vi "Pockels Cal-Write meas AI to sys config.vi"(8 "error in (no error)":errorcluster) -> (0 "error out":errorcluster)   [LabVIEW 2013]
uses:
  Typedefs/HW config states enum.ctl
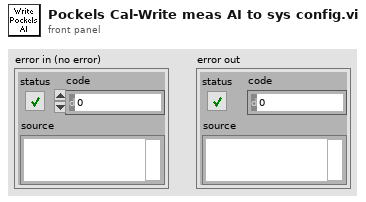
[diagram p1: front panel]
types:
  T1 = typedef "HW config states enum.ctl" = enum16{"Load from file", "Save to file", "Write all", "Read all", "Write XY stage settings", "Write DAQ FPGA settings", "Write Control FPGA settings", "Write Phys Channels", "Clear", "Compare from file"}
  T2 = typedef "Sys Configuration.ctl" = cluster{"XY Stage":T3, "DAQ FPGA":T4, "Control system":T8, "Encoder":T9, "DAQmx Chan":T10, "Computer MAC address":string, "Cam VidRec":T11, "Externalise Triggers":bool, "Laser wavelength (nm)":dbl}
  T3 = typedef "XY Stage config cluster.ctl" = cluster{"COM port":refnum<visa-resource-name>, "XY stage available":bool}
  T4 = typedef "DAQ FPGA config cluster.ctl" = cluster{"Ref":T5, "Target":T6, "Clock Freq (MHz) ":dbl, "input card type":T7, "Samples Wait after Trigger":u16, "AOD fill":u16, "StartupDelay":i32, "Slip Cycle (clock cycles)":u32, "Add Cycle":bool}
  T5 = typedef "FPGA Ref.ctl" = refnum<k20>
  T6 = typedef "nirio_resource_hc.ctl" = tag
  T7 = typedef "FPGA input type AC-DC.ctl" = enum16{"AC Card", "DC Card"}
  T8 = typedef "CTRL system config cluster.ctl" = cluster{"Ethernet opened":bool, "Ethernet Port":u32, "Ctrl FPGA available":bool, "Ctrl FPGA Clock (MHz)":dbl, "Ctrl system MAC address":string, "Control system.Network adapter name":string, "AOD 1 Amplitude":i16, "AOD 2 Amplitude":i16, "AOD 3 Amplitude":i16, "AOD 4 Amplitude":i16, "Data Time Interval (ns)":dbl, "T0 (ns)":dbl, "Ta (ns)":dbl}
  T9 = typedef "Encoder config cluster.ctl" = cluster{"IP address":string, "Port":u16, "Encoder available":bool, "Wheel radius (cm)":dbl}
  T10 = typedef "DAQmx physical channels cluster.ctl" = cluster{"Pockels AO":tag, "Hard shutter AO":tag, "PMT AOs":tag, "Power meter AI":tag}
  T11 = typedef "Cam VidRec HW config setup cluster.ctl" = cluster{"DO flag-Video record":tag, "DO flag-Trial start":tag, "VidRec available":bool}
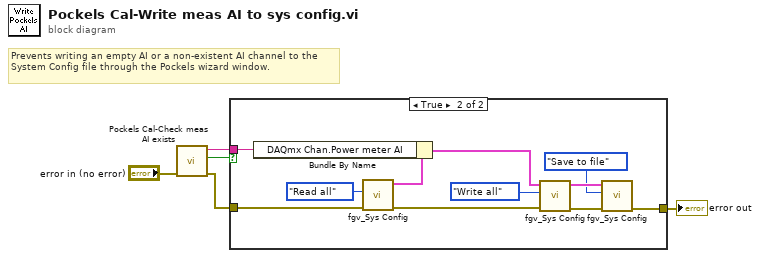
[diagram p0: block diagram]
diagram:
  # "Prevents writing an empty AI or a non-existent AI channel to the System Config file through the Pockels wizard window."
  n1 = call "Pockels Cal-Check meas AI exists.vi"("error in (no error)"="error in (no error)") -> ("error out"=w5:errorcluster, "Power-meter meas. AI channel exists"=w1:bool, "Power meter AI (dupl)"=w2:tag)  [unwired: 8 in]
  n2 = case shown="True" w1 {
    tunnel: w2 -> [_ w9]
    tunnel: w5 -> [w6 w8]
    tunnel: [w6 w7] -> w3
    frame False {
    }
    frame True {
      n3 = call "fgv_Sys Config.vi"("error in (no error)"=w8, "Function"=HW_config_states_enum."Read all") -> ("error out"=w17:errorcluster, "System Config out"=w12:T2)  [unwired: 8 in]
      n4 = Bundle By Name(cluster=w12, "DAQmx Chan.Power meter AI"=w9) -> (w13:T2)
      n5 = call "fgv_Sys Config.vi"("error in (no error)"=w17, "Function"=HW_config_states_enum."Write all", "System Config in"=w13) -> ("error out"=w16:errorcluster, "System Config out"=w15:T2)  [unwired: 7 in]
      n6 = call "fgv_Sys Config.vi"("error in (no error)"=w16, "Function"=HW_config_states_enum."Save to file", "System Config in"=w15) -> ("error out"=w7:errorcluster)  [unwired: 7 in, 1 out]
    }
  }
  "error out" <- w3
